vi "Handle getAll.vi"(8 "error in (no error)":errorcluster, 11 "Instrument.Framework-Template in":refnum<class "Instrument.Framework-Template.lvclass">) -> (0 "error out":errorcluster, 2 "getAll":variant, 3 "Instrument.Framework-Template out":refnum<class "Instrument.Framework-Template.lvclass">)   [LabVIEW 2019, in "Instrument.Framework-Template.lvclass"]
uses:
  Instrument.Framework-Template.lvclass
  Instrument.Framework-Template.lvclass/Instrument.Framework-Template.ctl
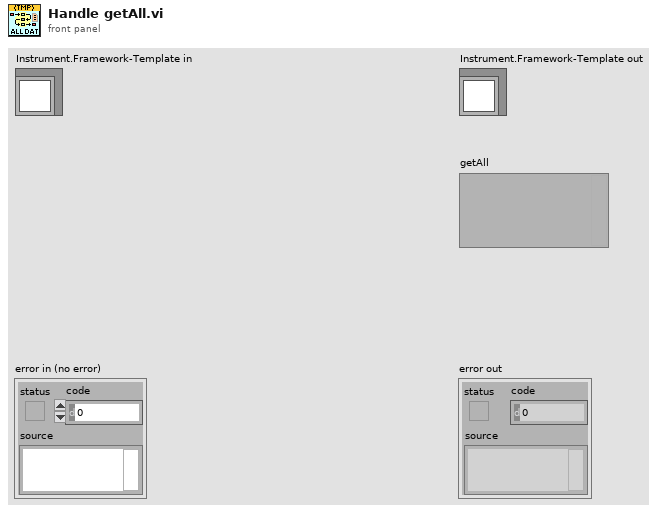
[diagram p1: front panel]
types:
  T1 = typedef "Instrument.Framework-Template.lvclass/Instrument.Framework-Template.getAll--Cluster.ctl" = cluster{"Levy 1":dbl, "Logger SMO":dbl, "SMO Boolean":bool, "SMO String":string}
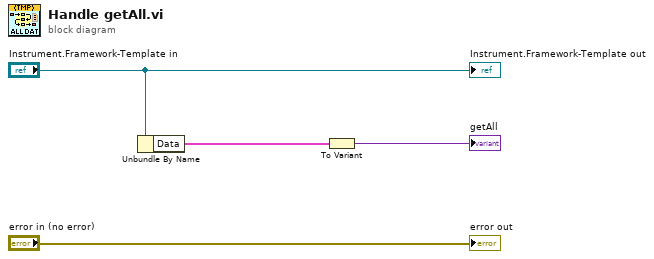
[diagram p0: block diagram]
diagram:
  n1 = Unbundle By Name("Instrument.Framework-Template in") -> ("Data"=w1:T1)
  n2 = To Variant(anything=w1) -> (Variant=→"getAll":variant)
  "error out" <- "error in (no error)"
  "Instrument.Framework-Template out" <- "Instrument.Framework-Template in"
